vi "Check license file.vi"(8 "error in (no error)":errorcluster, 10 "prefix text":string="tctechinc", 11 "file path":path) -> (0 "error out":errorcluster, 2 "valid?":bool, 3 "file path out":path)   [LabVIEW 2016]
doc: "Check the license file located in the assigned <b>file path</b> by the information of local MAC address and the <b>prefix text</b>. When the license file was generate by the same MAC address as local and same <b>prefix text</b> as assigned to the license generator. The VI return TRUE to the <b>valid?</b> sign. Error will occur when no license file or license file is invalid."
uses:
  <vilib>/Utility/error.llb/Error Cluster From Error Code.vi
  <vilib>/ErrorRing/Error Ring.xnode
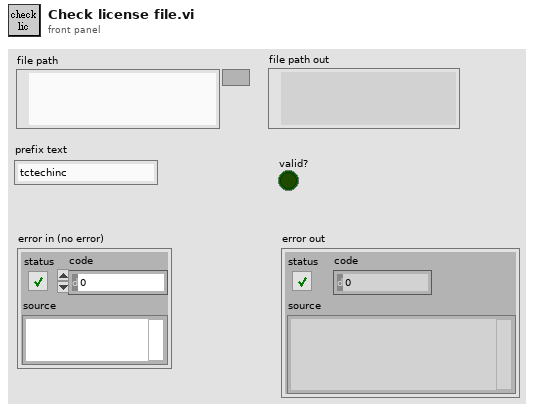
[diagram p1: front panel]
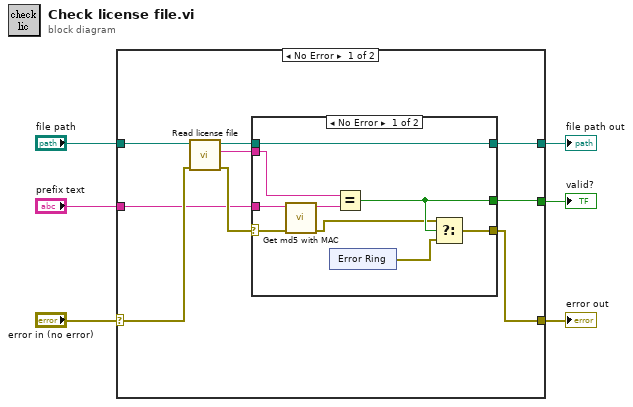
[diagram p0: block diagram]
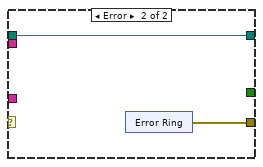
[diagram p2: hidden frame]
diagram:
  n1 = case shown="No Error" "error in (no error)" {
    selector: "error in (no error)" -> [w14 w38]
    tunnel: "prefix text" -> [w12 _]
    tunnel: "file path" -> [w15 w37]
    tunnel: [w9 w38] -> w3
    tunnel: [w10 _] -> w2
    tunnel: [w7 w37] -> w1
    frame No Error {
      n2 = call "Read license file.vi"("error in (no error)"=w14, "file path"=w15) -> ("error out"=w13:errorcluster, "MD5 Message Digest"=w11:string, "file path out"=w8:path)  [unwired: 7 in]
      n3 = case shown="No Error" w13 {
        selector: w13 -> [w23 _]
        tunnel: w12 -> [w24 _]
        tunnel: w11 -> [w21 _]
        tunnel: [w19 _] -> w10
        tunnel: [w17 w30] -> w9
        tunnel: w8 -> [w20 w31]
        tunnel: [w20 w31] -> w7
        frame No Error {
          n4 = call "Get md5 with MAC.vi"("error in (no error)"=w23, "prefix text"=w24) -> ("error out"=w18:errorcluster, "MD5 Message Digest"=w22:string)  [unwired: 8 in]
          n5 = xnode "Error Ring"() -> ("error out"=w16:errorcluster)
          n6 = Equal?(x=w21, y=w22) -> (x = y?=w19:bool)
          n7 = Select(t=w18, s=w19, f=w16) -> (s? t:f=w17:errorcluster)
        }
        frame Error {
          n8 = xnode "Error Ring"() -> ("error out"=w30:errorcluster)
        }
      }
    }
    frame Error {
    }
  }
  "error out" <- w3
  "valid?" <- w2
  "file path out" <- w1
